vi "Drive_Loop_Follow_Camera.vi"(10 "Power Level #6":dbl, 11 "Drive Loop Cluster":T1) -> ()   [LabVIEW 2016]
doc: "Help file written by FRC Team 836 - The RoboBees\n\nThis VI writes the \"Follow Camera\" command and power level #6 to the Drive Command RT FIFO in the Drive Loop Cluster.\n\nThe RT FIFO has to be initialized using the \"Drive_Loop_Initialize_w_Help\" VI"
uses:
  <userlib>/836-Libraries/Drive/Drive_Code/Drive_Code_Support/Drive_Code_Bundle.ctl
  <userlib>/836-Libraries/Drive/Drive_Code/Drive_Code_Support/Sensor_Cluster.ctl
  <userlib>/836-Libraries/Drive/Drive_Code/Drive_Code_Support/Camera_Cluster.ctl
  <userlib>/836-Libraries/Drive/Drive_Code/Drive_Code_Support/Drive_Code_Notifier.ctl
  <userlib>/836-Libraries/Drive/Drive_Code/Drive_Code_Support/Drive_Code_Command.ctl
  <userlib>/836-Libraries/Drive/Drive_Code/Logging_Data.ctl
  <userlib>/836-Libraries/Drive/Drive_Code/Drive_Code_Support/Drive_Code_PID_Bundle.ctl
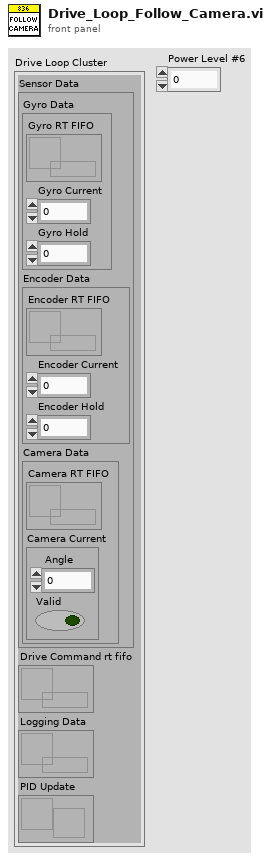
[diagram p1: front panel]
types:
  T1 = typedef "Drive_Code_Bundle.ctl" = cluster{"Sensor Data":T2, "Drive Command rt fifo":refnum<k33>, "Logging Data":refnum<k33>, "PID Update":refnum<notifier>}
  T2 = typedef "Sensor_Cluster.ctl" = cluster{"Gyro Data":cluster{"Gyro RT FIFO":refnum<k33>, "Gyro Current":dbl, "Gyro Hold":dbl}, "Encoder Data":cluster{"Encoder RT FIFO":refnum<k33>, "Encoder Current":dbl, "Encoder Hold":dbl}, "Camera Data":cluster{"Camera RT FIFO":refnum<k33>, "Camera Current":T3}}
  T3 = typedef "Camera_Cluster.ctl" = cluster{" Angle":dbl, "Valid":bool}
  T4 = typedef "Drive_Code_Command.ctl" = enum16{"Do Nothing", "Manual", "Drive Continuous", "Turn", "Drive Distance", "Hold Position", "Hold Yaw", "Follow Camera", "Turn to Camera", "Approach Camera"}
  T5 = typedef "Drive_Code_Notifier.ctl" = cluster{"Command":T4, "Parameter A":dbl, "Parameter B":dbl, "Parameter C":dbl, "Absolute?":bool}
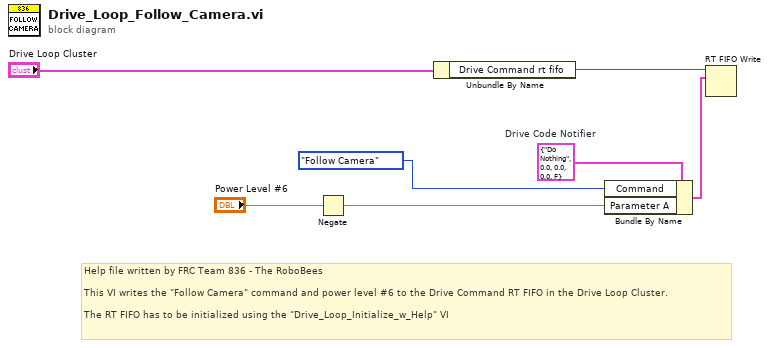
[diagram p0: block diagram]
diagram:
  w1 = T5 {"Command"=enum."Do Nothing", "Parameter A"=0.0, "Parameter B"=0.0, "Parameter C"=0.0, "Absolute?"=FALSE}  # Drive Code Notifier
  # "Help file written by FRC Team 836 - The RoboBees\n\nThis VI writes the \"Follow Camera\" command and power level #6 to the Drive Command RT FIFO in the Drive Loop Cluster.\n\nThe RT FIFO has to be initialized using the \"Drive_Loop_Initialize_w_Help\" VI"
  n1 = Negate(x="Power Level #6") -> (-x=w4:dbl)
  n2 = Unbundle By Name("Drive Loop Cluster") -> ("Drive Command rt fifo"=w6:refnum<k33>)
  n3 = Bundle By Name(cluster=w1, "Command"=Drive_Code_Command."Follow Camera", "Parameter A"=w4) -> (w7:T5)
  n4 = RT FIFO Write(0:w6, 1:w7) -> ()  [unwired: 3 in, 4 out]
